vi "Spectral Transform.vi"(0 "Input Signal":dbl[](array[numeric])) -> (1 "STFT":dbl[][](array[numeric]), 2 "Frequency Axis Scale Factor":dbl)   [LabVIEW 2014, in "Melody Extraction.lvlib"]
uses:
  Melody Extraction.lvlib
  <vilib>/Analysis/4window.llb/windowTd.ctl
  dt_global.vi
  <vilib>/gmath/NI_Gmath.lvlib
  <vilib>/Analysis/NI_AALPro.lvlib
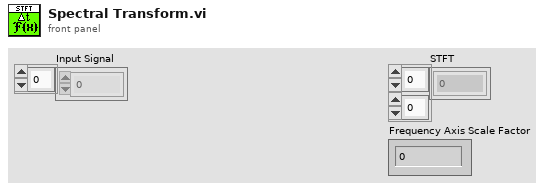
[diagram p1: front panel]
types:
  T1 = cluster{"force freq bins to power of 2?":bool, "exclude Nyquist frequency?":bool}
  T2 = typedef "NI_AALPro.lvlib/windowTd.ctl" = u32
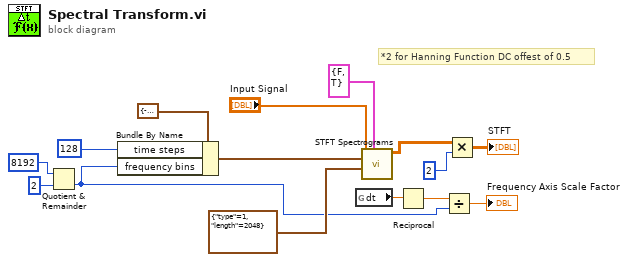
[diagram p0: block diagram]
diagram:
  # "*2 for Hanning Function DC offest of 0.5"
  n1 = Quotient & Remainder(x=8192 ("time steps"), y=2) -> (floor(x/y)=w5:i32)  [unwired: 1 out]
  n2 = Bundle By Name(cluster=cluster{"time steps":i32, "frequency bins":i32} {"time steps"=-1, "frequency bins"=512} ("time-freq sampling info"), "time steps"=128, "frequency bins"=w5) -> (w11:cluster{"time steps":i32, "frequency bins":i32})
  n3 = global read "dt_global.vi" "dt"() -> (w7:dbl)
  n4 = call <vilib>:"STFT Spectrograms.vi"("time-freq config"=T1 {"force freq bins to power of 2?"=FALSE, "exclude Nyquist frequency?"=TRUE}, "window info"=cluster{"type":T2, "length":i32} {"type"=1, "length"=2048}, "time-freq sampling info"=w11, "X"="Input Signal") -> ("STFT Spectrogram {X}"=w3:dbl[][])  [unwired: 6 in, 1 out]
  n5 = Reciprocal(x=w7) -> (1/x=w6:dbl)
  n6 = Divide(x=w6, y=w5) -> (x/y=→"Frequency Axis Scale Factor":dbl)
  n7 = Multiply(x=w3, y=2) -> (x*y=→"STFT":dbl[][])
